vi "ini path.vi"() -> ()   [LabVIEW 2010]
panel:
  out "ini path":path
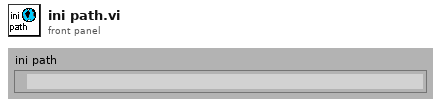
[diagram p1: front panel]
diagram:
